vi "XYStage.ReadPosition.vi"(8 "error in (no error)":errorcluster, 11 "XYStage":refnum<class "XYStage.lvclass">) -> (0 "error out":errorcluster, 1 "Counts out":T1, 2 "Position":T2, 3 "XYStage out":refnum<class "XYStage.lvclass">)   [LabVIEW 2015, in "XYStage.lvclass"]
doc: "---------------------------------------------------------------\nJKI State Machine Objects™\nhttp://jki.net/state-machine-objects/\nCopyright (C) 2005-2015, JKI <info@jki.net>\nALL RIGHTS RESERVEDJKI State Machine Objects (SMO) 1.0.0.5\nJKI - JKI\nCopyright (c) 2016, JKI"
uses:
  XYStage.lvclass
  Typedefs/(real)Coords--Cluster.ctl
  Typedefs/(counts)Coords--Cluster.ctl
panel:
  # "For instructions on how to use the JKI State Machine Objects, examples and video tutorials, visit:\nhttp://jki.net/state-machine-objects/\n\nJKI State Machine Objects™\nhttp://jki.net/state-machine-objects/\nCopyright (C) 2005-2015, JKI <info@jki.net>\nALL RIGHTS RESERVED"
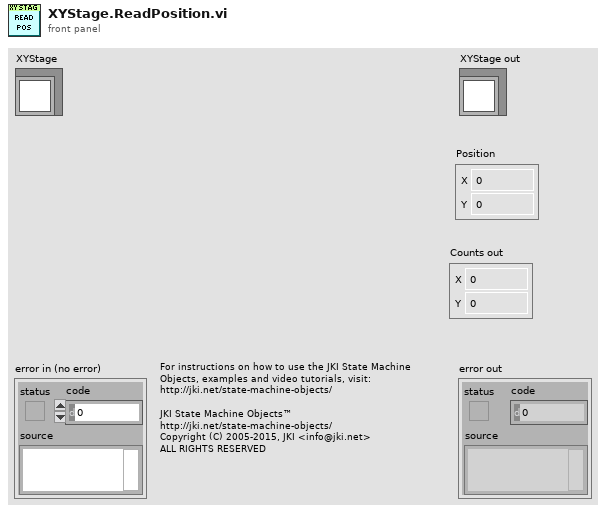
[diagram p1: front panel]
types:
  T1 = typedef "XYStage.lvclass/(counts)Coords--Cluster.ctl" = cluster{"X":i32, "Y":i32}
  T2 = typedef "XYStage.lvclass/(real)Coords--Cluster.ctl" = cluster{"X":dbl, "Y":dbl}
  T3 = typedef "XYStage.lvclass/TargetPositions--Cluster.ctl" = cluster{"Coords":T2, "Counts":T1}
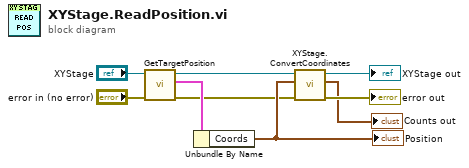
[diagram p0: block diagram]
diagram:
  n1 = call "GetTargetPosition.vi"("error in (no error)"="error in (no error)", "XYStage"="XYStage") -> ("error out"=w1:errorcluster, "Target"=w7:T3, "XYStage out"=w3:refnum<class "XYStage.lvclass">)  [unwired: 7 in]
  n2 = Unbundle By Name(w7) -> ("Coords"=w2:T2)
  "Position" <- w2
  n3 = call-dynamic "XYStage.ConvertCoordinates.vi"("error in (no error)"=w1, "Real Units Coords"=w2, "XYStage in"=w3) -> ("error out"=→"error out":errorcluster, "Counts out"=→"Counts out":T1, "XYStage out"=→"XYStage out":refnum<class "XYStage.lvclass">)  [unwired: 5 in, 1 out]
